vi "waveform_chart.vi"() -> ()   [LabVIEW 2020]
panel:
  out "Waveform Chart":dbl(graph)
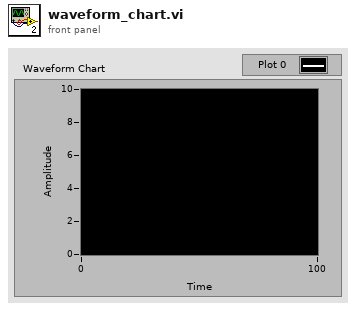
[diagram p1: front panel]
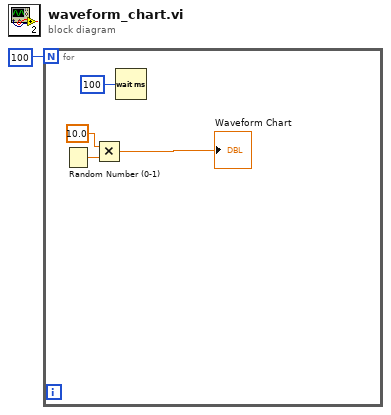
[diagram p0: block diagram]
diagram:
  n1 = for {
    N: 100 -> [_]
    n2 = Random Number (0-1)() -> (number: 0 to 1=w4:dbl)
    n3 = Multiply(x=10.0, y=w4) -> (x*y=→"Waveform Chart":dbl)
    n4 = Wait (ms)(milliseconds to wait=u32 100) -> ()  [unwired: 1 out]
  }
